vi "Stepper Write.vi"(6 "Set Acceleration (0 to disable)":i16, 7 "Stepper #":u8, 8 "error in":errorcluster, 9 "Set Speed (Steps per Second)":i16=100, 10 "# of Steps to Move":i16, 11 "Arduino Resource":T1={"VISA resource"="", "Board Type"=enum."Uno", "Connection Type"=enum."USB / Serial", "Bytes Per Packet (15)"=15}) -> (0 "error out":errorcluster, 3 "Arduino Resource Out":T1={"VISA resource"="", "Board Type"=enum."Uno", "Connection Type"=enum."USB / Serial", "Bytes Per Packet (15)"=15})   [LabVIEW 2011, in "LabVIEW Interface for Arduino.lvlib"]
doc: "Specify the speed and number of steps to move the stepper motor. Optionally, specify acceleration in steps per second per second."
uses:
  <vilib>/LabVIEW Interface for Arduino/LabVIEW Interface for Arduino.lvlib
  <vilib>/LabVIEW Interface for Arduino/Private/Type Defs/Arduino Resource.ctl
  <vilib>/LabVIEW Interface for Arduino/Private/Type Defs/Board Type.ctl
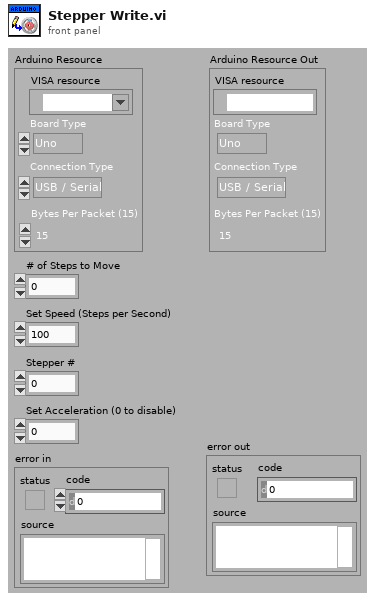
[diagram p1: front panel]
types:
  T1 = typedef "LabVIEW Interface for Arduino.lvlib/Arduino Resource.ctl" = cluster{"VISA resource":refnum<visa-resource-name>, "Board Type":T2, "Connection Type":enum8{"USB / Serial"}, "Bytes Per Packet (15)":u8}
  T2 = typedef "LabVIEW Interface for Arduino.lvlib/Board Type.ctl" = enum16{"Uno", "Dimuelanove w/Atmega 328", "Mega 2560"}
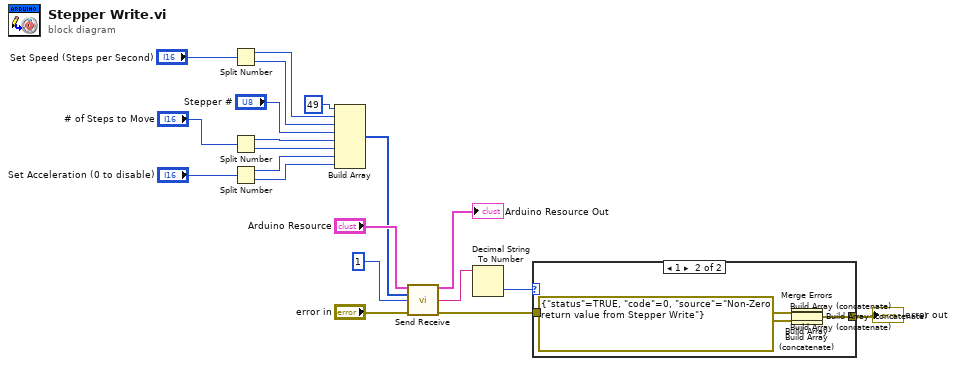
[diagram p0: block diagram]
diagram:
  n1 = Split Number(x="Set Speed (Steps per Second)") -> (hi(x)=w12:u8, lo(x)=w11:u8)
  n2 = Split Number(x="# of Steps to Move") -> (hi(x)=w9:u8, lo(x)=w8:u8)
  n3 = Split Number(x="Set Acceleration (0 to disable)") -> (hi(x)=w6:u8, lo(x)=w5:u8)
  n4 = Build Array(u8 49, w12, w11, "Stepper #", w9, w8, w6, w5) -> (w16:u8[])
  n5 = call <vilib>:"Send Receive.vi"("Arduino Resource"="Arduino Resource", "Data"=w16, "Bytes To Read (0)"=u8 1, "error in"="error in") -> ("Arduino Resource"=→"Arduino Resource Out":T1, "Read Buffer"=w1:string, "error out"=w2:errorcluster)  [unwired: 9 in]
  n6 = Decimal String To Number(string=w1) -> (number=w4:i32)  [unwired: 2 in, 1 out]
  n7 = case shown="1" w4 {
    tunnel: w2 -> [w21 w29]
    tunnel: [w21 w28] -> w3
    frame 0, Default {
    }
    frame 1 {
      n8 = Build Array(w29, errorcluster {"status"=TRUE, "code"=0, "source"="Non-Zero return value from Stepper Write"} ("error in")) -> (w26:errorcluster[])
      n9 = Build Array (concatenate)(w26) -> (w25:errorcluster[])
      n10 = Build Array (concatenate)(w25) -> (w24:errorcluster[])
      n11 = Build Array (concatenate)(w24) -> (w23:errorcluster[])
      n12 = Build Array (concatenate)(w23) -> (w22:errorcluster[])
      n13 = Merge Errors(w22) -> (w28:errorcluster)
    }
  }
  "error out" <- w3
